vi "InitializeCurrentMeters.vi"(8 "Error In":errorcluster, 10 "Keithley 6482":T1, 11 "Keithley 6485":T2) -> (0 "Error Out":errorcluster, 3 "Current Meters Out":refnum<visa-resource-name>[](array[refnum]))   [LabVIEW 2012]
uses:
  Keithley6485Configuration.ctl
  Keithley6482Configuration.ctl
  libs/LV-Utilities/LV-Utilities.lvlib
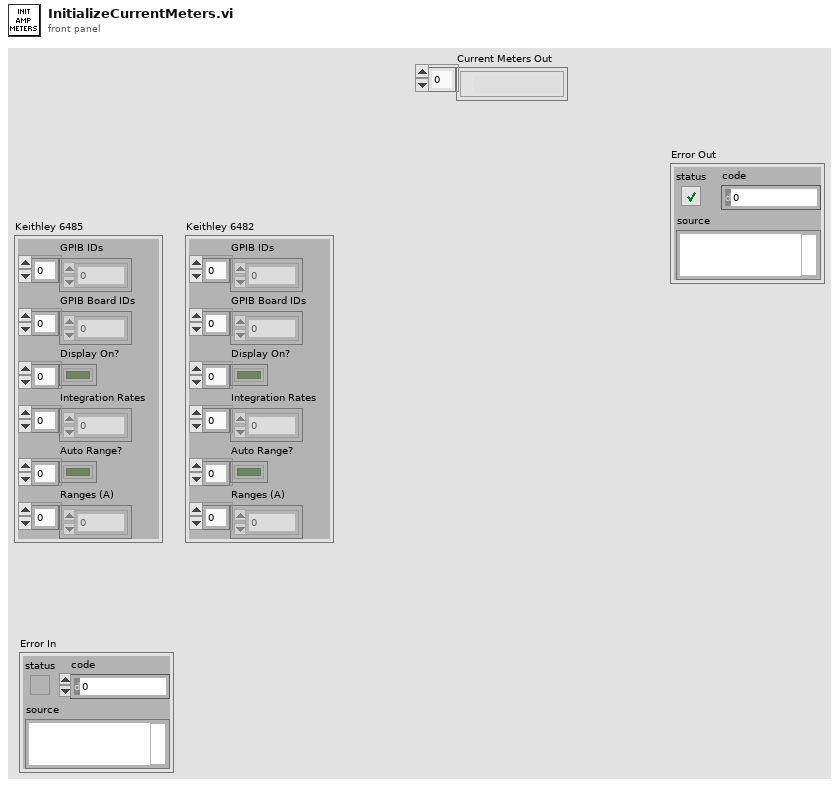
[diagram p1: front panel]
types:
  T1 = typedef "Keithley6482Configuration.ctl" = cluster{"GPIB IDs":u8[], "GPIB Board IDs":u8[], "Display On?":bool[], "Integration Rates":dbl[], "Auto Range?":bool[], "Ranges (A)":dbl[]}
  T2 = typedef "Keithley6485Configuration.ctl" = cluster{"GPIB IDs":u8[], "GPIB Board IDs":u8[], "Display On?":bool[], "Integration Rates":dbl[], "Auto Range?":bool[], "Ranges (A)":dbl[]}
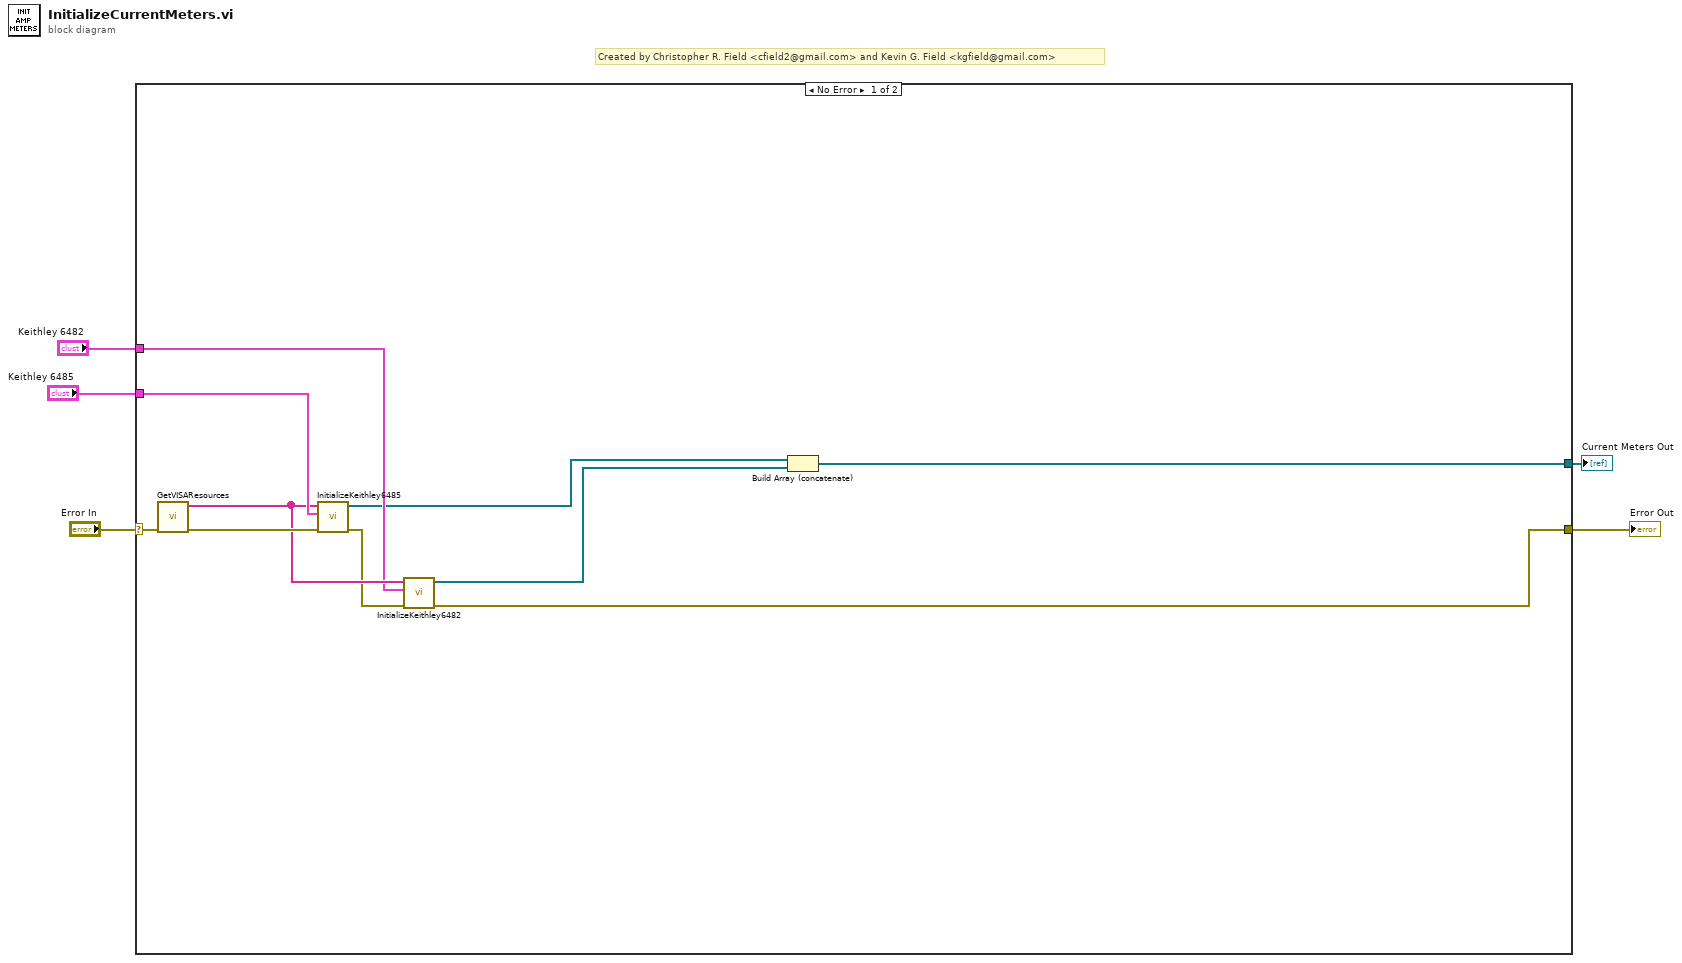
[diagram p0: block diagram]
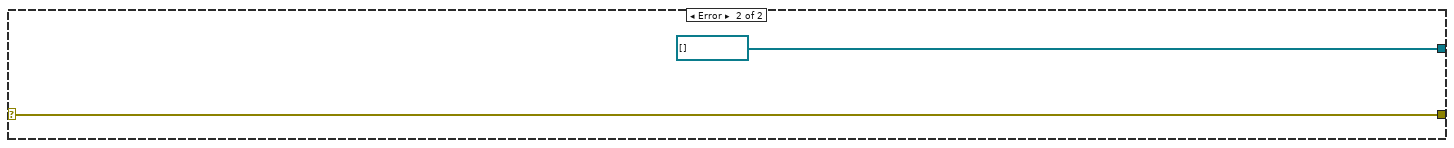
[diagram p2: hidden frame]
diagram:
  # "Created by Christopher R. Field <cfield2@gmail.com> and Kevin G. Field <kgfield@gmail.com>"
  n1 = case shown="No Error" "Error In" {
    selector: "Error In" -> [w15 w17]
    tunnel: "Keithley 6485" -> [w13 _]
    tunnel: "Keithley 6482" -> [w10 _]
    tunnel: [w9 w17] -> w2
    tunnel: [w6 refnum<visa-resource-name>[] []] -> w1
    frame No Error {
      n2 = call "GetVISAResources.vi"("Error In"=w15) -> ("Error Out"=w14:errorcluster, "VISA Resources"=w12:string[])  [unwired: 9 in]
      n3 = call "InitializeKeithley6485.vi"("Error In"=w14, "Keithley 6485"=w13, "VISA Resources"=w12) -> ("Error Out"=w11:errorcluster, "Keithley 6485 Out"=w8:refnum<visa-resource-name>[])  [unwired: 7 in]
      n4 = call "InitializeKeithley6482.vi"("Error In"=w11, "Keithley 6482"=w10, "VISA Resources"=w12) -> ("Error Out"=w9:errorcluster, "Keithley 6482 Out"=w7:refnum<visa-resource-name>[])  [unwired: 7 in]
      n5 = Build Array (concatenate)(w8, w7) -> (w6:refnum<visa-resource-name>[])
    }
    frame Error {
    }
  }
  "Error Out" <- w2
  "Current Meters Out" <- w1
